vi "CLD 5 Parse Config Data File Solution.vi"(8 "error in (no error)":errorcluster, 10 "Array In":T1[][](array[typedef])=[[{"Numeric"=2.25, "Boolean"=FALSE, "String"="One"}, {"Numeric"=1.35, "Boolean"=TRUE, "String"="Two"}, {"Numeric"=1.5, "Boolean"=FALSE, "String"="Three"}, {"Numeric"=1.0, "Boolean"=TRUE, "String"="Four"}], [{"Numeric"=2.0, "Boolean"=TRUE, "String"="Five"}, {"Numeric"=0.75, "Boolean"=FALSE, "String"="Six"}, {"Numeric"=0.9, "Boolean"=TRUE, "String"="Seven"}, {"Numeric"=0.75, "Boolean"=FALSE, "String"="Eight"}]], 11 "Get/Set":enum16{"Get", "Set"}(ring)) -> (0 "error out":errorcluster, 2 "Array Out":T1[][](array[typedef]))   [LabVIEW 2025]
doc: "CLD 5 exercise. Use of Configuration File VI's to read and write to file and to a data cluster. The data uses a two dimensional configuration, this must be accounted for in the data structure."
uses:
  CLD 5 Data Cluster.ctl
  <vilib>/Utility/config.llb/Read Key (Double).vi
  <vilib>/Utility/config.llb/Read Key (Boolean).vi
  <vilib>/Utility/config.llb/Read Key (String).vi
  <vilib>/Utility/config.llb/Read Key (I32).vi
  <vilib>/Utility/config.llb/Write Key (Double).vi
  <vilib>/Utility/config.llb/Write Key (Boolean).vi
  <vilib>/Utility/config.llb/Write Key (String).vi
  <vilib>/Utility/config.llb/Write Key (I32).vi
  <vilib>/Utility/config.llb/NI_LVConfig.lvlib
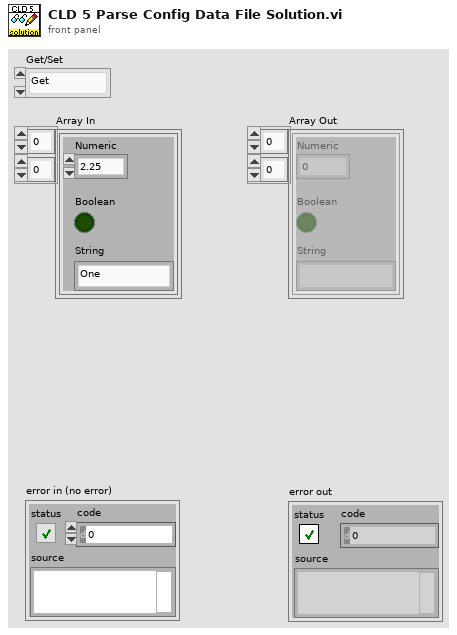
[diagram p1: front panel]
types:
  T1 = typedef "CLD 5 Data Cluster.ctl" = cluster{"Numeric":dbl, "Boolean":bool, "String":string}
  T2 = typedef "NI_LVConfig.lvlib/Config Data RefNum.ctl" = refnum<k1>
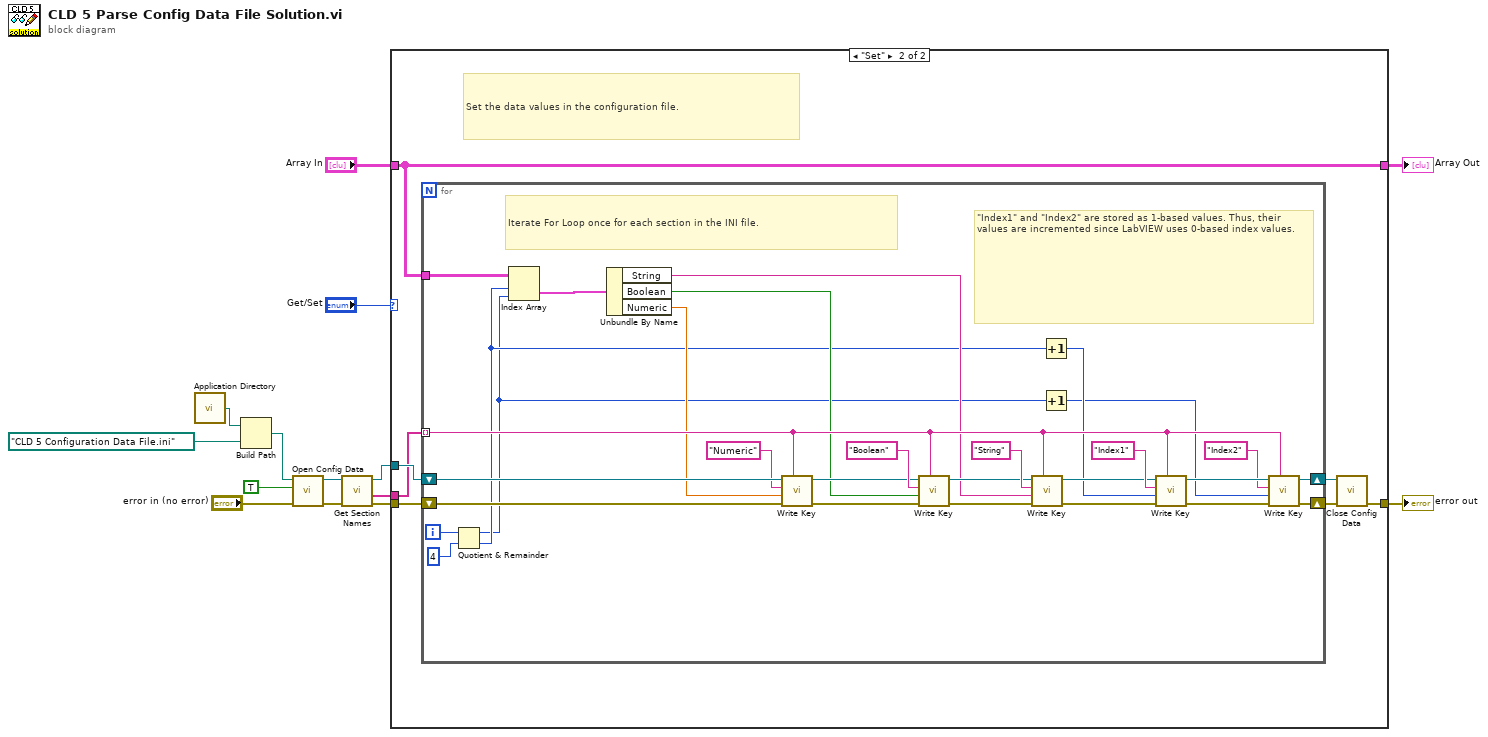
[diagram p0: block diagram]
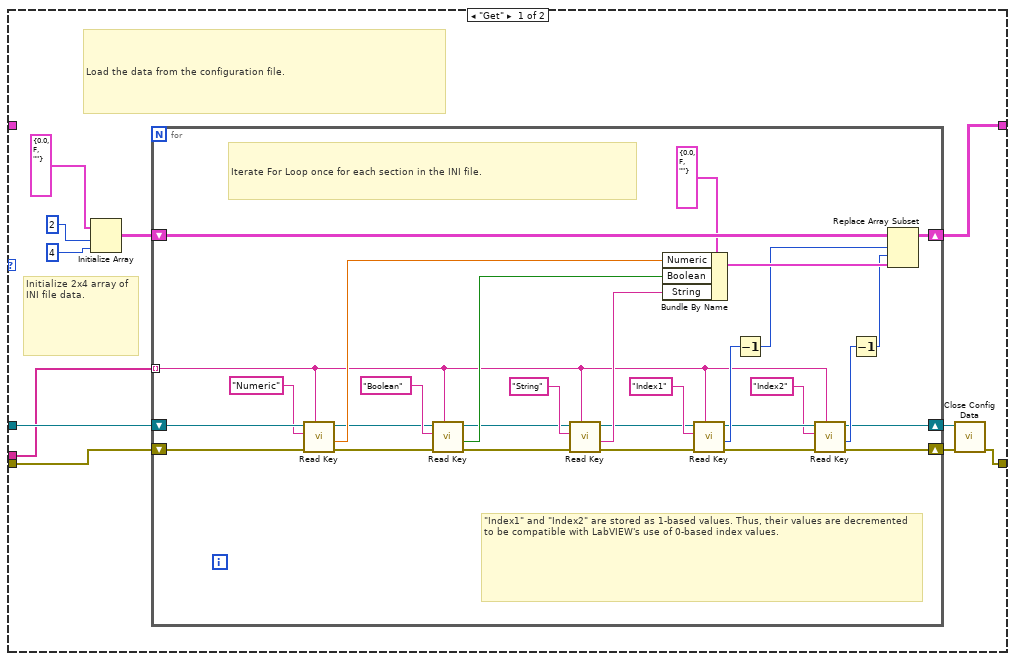
[diagram p2: hidden frame]
diagram:
  n1 = call <vilib>:"Application Directory.vi"() -> ("Application Directory"=w6:path)
  n2 = Build Path(base path=w6, name or relative path=path "CLD 5 Configuration Data File.ini") -> (appended path=w13:path)
  n3 = call <vilib>:"Open Config Data.vi"("error in (no error)"="error in (no error)", "create file if necessary (T)"=TRUE, "configuration file path"=w13) -> ("error out"=w9:errorcluster, "refnum"=w4:T2)  [unwired: 6 in, 1 out]
  n4 = call <vilib>:"Get Section Names.vi"("error in (no error)"=w9, "refnum"=w4) -> ("error out"=w5:errorcluster, "section names"=w2:string[], "refnum out"=w3:T2)  [unwired: 7 in]
  n5 = case shown="\"Set\"" "Get/Set" {
    tunnel: w5 -> [w25 w61]
    tunnel: w3 -> [w24 w60]
    tunnel: "Array In" -> [_ w55]
    tunnel: [w21 w57] -> w7
    tunnel: [w15 w55] -> w1
    tunnel: w2 -> [w20 w56]
    frame "Get" {
      # "Initialize 2x4 array of INI file data."
      # "Load the data from the configuration file."
      n6 = Initialize Array(T1 {"Numeric"=0.0, "Boolean"=FALSE, "String"=""} ("Array"), 2 ("dimension size"), 4 ("dimension size")) -> (w16:T1[][])
      n7 = for {
        shift-right: [w27] -> w23
        shift-left: w25 -> [w54]
        shift-right: [w26] -> w22
        shift-left: w24 -> [w53]
        tunnel: w20 -> [w30] mode=indexing
        shift-right: [w50] -> w15
        shift-left: w16 -> [w51]
        # "\"Index1\" and \"Index2\" are stored as 1-based values. Thus, their values are decremented to be compatible with LabVIEW's use of 0-based index values."
        # "Iterate For Loop once for each section in the INI file."
        n8 = call-poly <vilib>:"Read Key.vi"("section"=w30, "error in (no error)"=w54, "key"="Numeric", "refnum"=w53) -> ("error out"=w44:errorcluster, "value"=w47:dbl, "refnum out"=w45:T2)  [unwired: 4 in, 1 out]
        n9 = call-poly <vilib>:"Read Key.vi"("section"=w30, "error in (no error)"=w44, "key"="Boolean", "refnum"=w45) -> ("error out"=w42:errorcluster, "value"=w43:bool, "refnum out"=w40:T2)  [unwired: 4 in, 1 out]
        n10 = call-poly <vilib>:"Read Key.vi"("section"=w30, "error in (no error)"=w42, "key"="String", "refnum"=w40) -> ("error out"=w37:errorcluster, "value"=w39:string, "refnum out"=w36:T2)  [unwired: 4 in, 1 out]
        n11 = Bundle By Name(cluster=T1 {"Numeric"=0.0, "Boolean"=FALSE, "String"=""} ("Array"), "Numeric"=w47, "Boolean"=w43, "String"=w39) -> (w48:T1)
        n12 = call-poly <vilib>:"Read Key.vi"("section"=w30, "error in (no error)"=w37, "key"="Index1", "refnum"=w36) -> ("error out"=w33:errorcluster, "value"=w35:i32, "refnum out"=w32:T2)  [unwired: 4 in, 1 out]
        n13 = Decrement(x=w35) -> (x-1=w34:i32)
        n14 = call-poly <vilib>:"Read Key.vi"("section"=w30, "error in (no error)"=w33, "key"="Index2", "refnum"=w32) -> ("error out"=w27:errorcluster, "value"=w29:i32, "refnum out"=w26:T2)  [unwired: 4 in, 1 out]
        n15 = Decrement(x=w29) -> (x-1=w28:i32)
        n16 = Replace Array Subset(array=w51, new element=w48, index (row)=w34, index (col)=w28) -> (w50:T1[][])
      }
      n17 = call <vilib>:"Close Config Data.vi"("error in (no error)"=w23, "refnum"=w22) -> ("error out"=w21:errorcluster)  [unwired: 8 in, 1 out]
    }
    frame "Set" {
      # "Set the data values in the configuration file."
      n18 = for {
        shift-right: [w74] -> w59
        shift-left: w61 -> [w90]
        shift-right: [w73] -> w58
        shift-left: w60 -> [w89]
        tunnel: w56 -> [w75] mode=indexing
        tunnel: w55 -> [w72]
        i -> [w70]
        # "\"Index1\" and \"Index2\" are stored as 1-based values. Thus, their values are incremented since LabVIEW uses 0-based index values."
        # "Iterate For Loop once for each section in the INI file."
        n19 = Quotient & Remainder(x=w70, y=4) -> (x-y*floor(x/y)=w64:i32, floor(x/y)=w65:i32)
        n20 = Index Array(array=w72, index (row)=w65, index (col)=w64) -> (element=w71:T1)
        n21 = Unbundle By Name(w71) -> ("String"=w66:string, "Boolean"=w67:bool, "Numeric"=w68:dbl)
        n22 = call-poly <vilib>:"Write Key.vi"("section"=w75, "error in (no error)"=w90, "value"=w68, "key"="Numeric", "refnum"=w89) -> ("error out"=w85:errorcluster, "refnum out"=w86:T2)  [unwired: 4 in, 1 out]
        n23 = call-poly <vilib>:"Write Key.vi"("section"=w75, "error in (no error)"=w85, "value"=w67, "key"="Boolean", "refnum"=w86) -> ("error out"=w84:errorcluster, "refnum out"=w82:T2)  [unwired: 4 in, 1 out]
        n24 = call-poly <vilib>:"Write Key.vi"("section"=w75, "error in (no error)"=w84, "value"=w66, "key"="String", "refnum"=w82) -> ("error out"=w80:errorcluster, "refnum out"=w79:T2)  [unwired: 4 in, 1 out]
        n25 = Increment(x=w65) -> (x+1=w63:i32)
        n26 = Increment(x=w64) -> (x+1=w62:i32)
        n27 = call-poly <vilib>:"Write Key.vi"("section"=w75, "error in (no error)"=w80, "value"=w63, "key"="Index1", "refnum"=w79) -> ("error out"=w78:errorcluster, "refnum out"=w77:T2)  [unwired: 4 in, 1 out]
        n28 = call-poly <vilib>:"Write Key.vi"("section"=w75, "error in (no error)"=w78, "value"=w62, "key"="Index2", "refnum"=w77) -> ("error out"=w74:errorcluster, "refnum out"=w73:T2)  [unwired: 4 in, 1 out]
      }
      n29 = call <vilib>:"Close Config Data.vi"("error in (no error)"=w59, "refnum"=w58) -> ("error out"=w57:errorcluster)  [unwired: 8 in, 1 out]
    }
  }
  "error out" <- w7
  "Array Out" <- w1
